vi "Two_neuron_oscillator_modulated.vi"() -> ()   [LabVIEW 2016]
uses:
  <vilib>/measure/NI_MABase.lvlib
panel:
  in  "frequency":dbl=0.625 format="%#_13g"
  out "W":T1(graph)
  in  "M":dbl[](array[numeric])=[1.0, 1.0, 1.0, -1.0, 1.0]
  in  "Simulation delay":u32=10
  out "Neurons":T2(graph)
  out "Viewer":T3={"NoPre"=[0, 2, 2], "Pre IDs"=[0, 1, 2, 1, 2], "W"=[1.0, 1.0, 1.0, -1.0, 1.0], "Current"=[1.0, 0.0, 0.0]}
  in  "stop":bool
  in  "Network AER Vectors":T3={"NoPre"=[0, 2, 2], "Pre IDs"=[0, 1, 2, 1, 2], "W"=[1.0, 1.0, 1.0, -1.0, 1.0], "Current"=[1.0, 0.0, 0.0]}
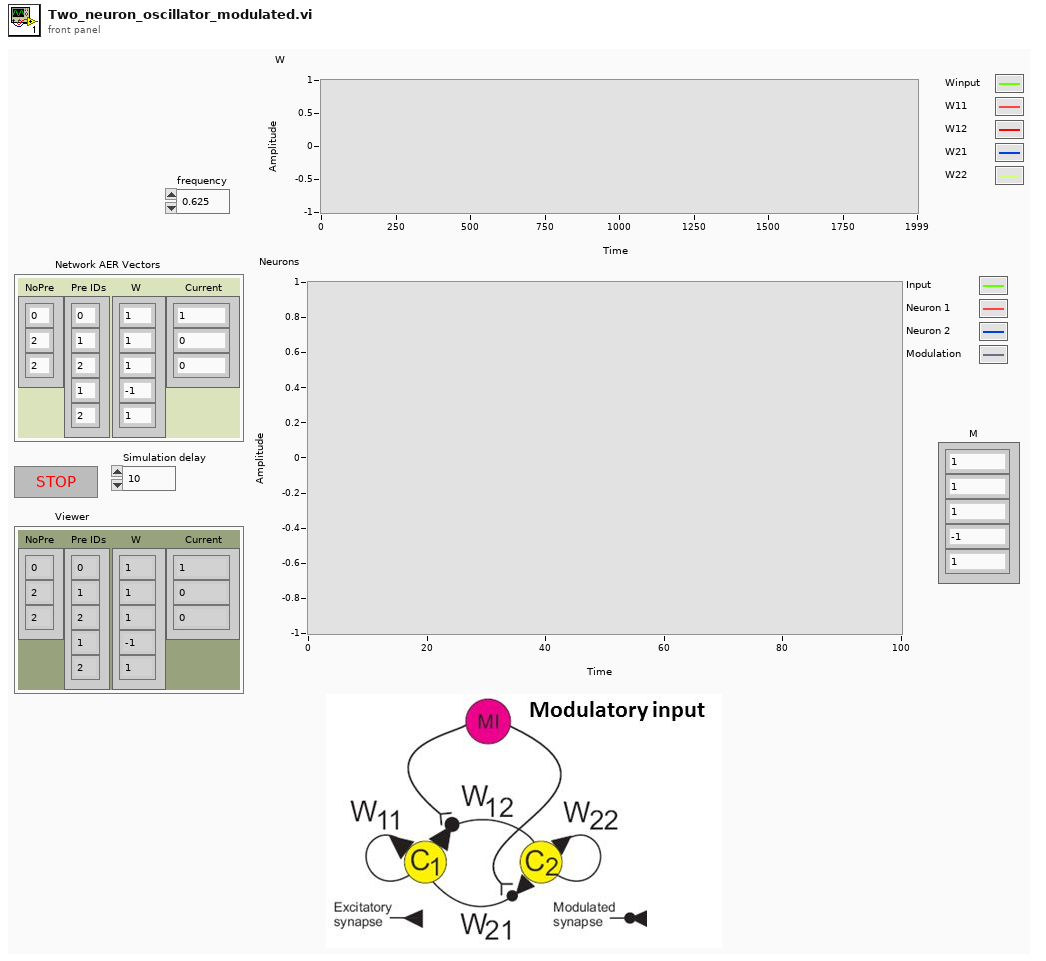
[diagram p1: front panel]
types:
  T1 = cluster{"W[0]":dbl, "W[1]":dbl, "W[2]":dbl, "W[3]":dbl, "W[4]":dbl}
  T2 = cluster{"Current[0]":dbl, "Current[1]":dbl, "Current[2]":dbl, "Current[3]":dbl}
  T3 = cluster{"NoPre":i32[], "Pre IDs":i32[], "W":dbl[], "Current":dbl[]}
  T4 = cluster{"[0]":dbl, "[1]":dbl, "[2]":dbl, "[3]":dbl}
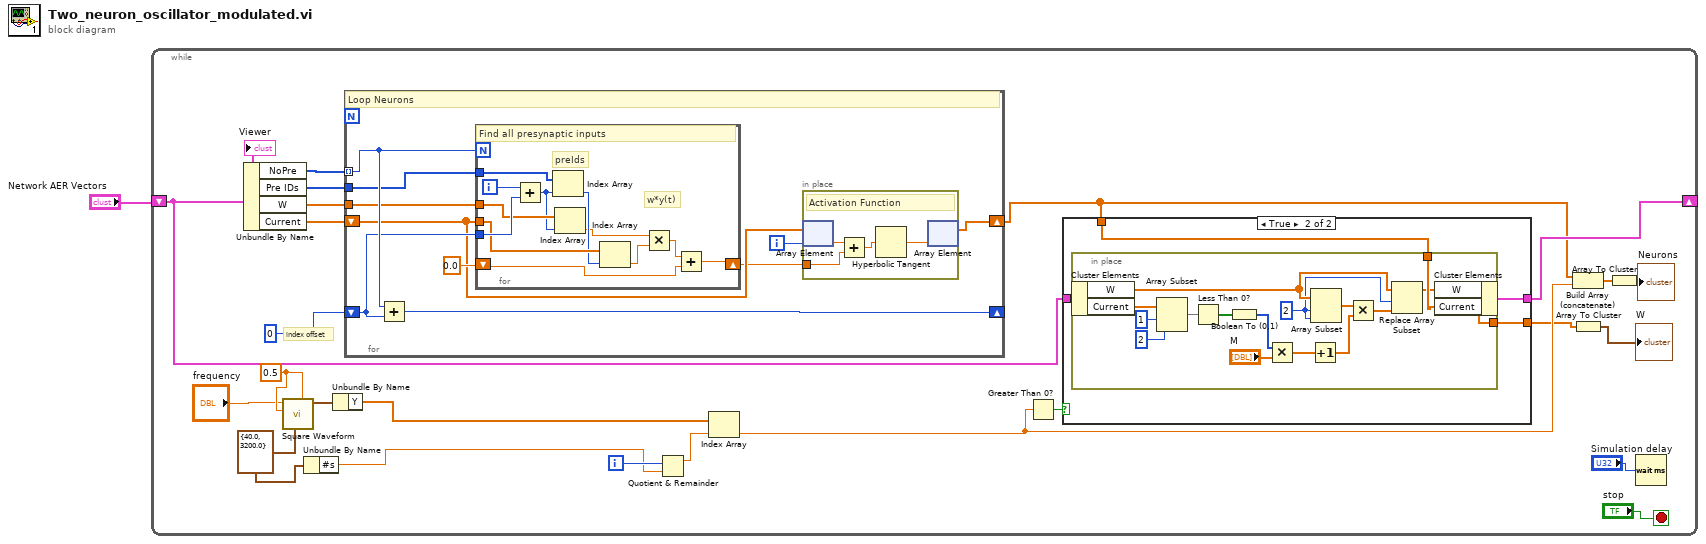
[diagram p0: block diagram]
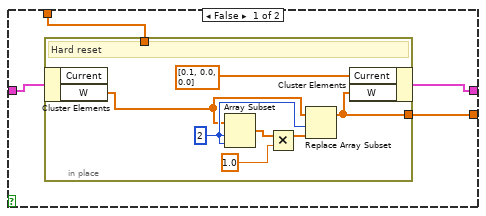
[diagram p2: hidden frame]
diagram:
  n1 = while {
    shift-right: [w11] -> _
    shift-left: "Network AER Vectors" -> [w13]
    i -> [w15]
    stop <- "stop" stop-if-true
    w7 = 0.5 ("offset")
    w6 = cluster{"Fs":dbl, "#s":dbl} {"Fs"=40.0, "#s"=3200.0} ("sampling info")
    # "index offset"
    n2 = Unbundle By Name(w13) -> ("NoPre"=w25:i32[], "Pre IDs"=w23:i32[], "W"=w22:dbl[], "Current"=w21:dbl[])
    n3 = call <vilib>:"Square Waveform.vi"("offset"=w7, "sampling info"=w6, "amplitude"=w7, "frequency"="frequency") -> ("signal out"=w5:waveform(dbl))  [unwired: 6 in, 1 out]
    n4 = Unbundle By Name(w6) -> ("#s"=w2:dbl)
    n5 = Unbundle By Name(w5) -> ("Y"=w3:dbl[])
    n6 = for {
      tunnel: w25 -> [w64] mode=indexing
      shift-right: [w65] -> _
      shift-left: 0 -> [w63]
      tunnel: w23 -> [w62]
      tunnel: w22 -> [w56]
      shift-right: [w57] -> w10
      shift-left: w21 -> [w60]
      i -> [w59]
      # "Loop Neurons"
      n7 = Add(x=w64, y=w63) -> (x+y=w65:i32)
      n8 = for {
        N: w64 -> [_]
        tunnel: w63 -> [w80]
        tunnel: w62 -> [w79]
        tunnel: w56 -> [w78]
        tunnel: w60 -> [w77]
        shift-right: [w73] -> w58
        shift-left: 0.0 -> [w71]
        i -> [w81]
        # "w*y(t)"
        # "preIds"
        # "Find all presynaptic inputs"
        n9 = Add(x=w81, y=w80) -> (x+y=w70:i32)
        n10 = Index Array(array=w79, index=w70) -> (element=w76:i32)
        n11 = Index Array(array=w78, index=w70) -> (element=w75:dbl)
        n12 = Index Array(array=w77, index=w76) -> (element=w74:dbl)
        n13 = Multiply(x=w75, y=w74) -> (x*y=w72:dbl)
        n14 = Add(x=w72, y=w71) -> (x+y=w73:dbl)
      }
      n15 = in-place {
        in-place-border: w58 -> [w69]
        # "Activation Function"
        n16 = in-place-array #1(w60, w59) -> (w67:dbl)
        n17 = Add(x=w67, y=w69) -> (x+y=w66:dbl)
        n18 = Hyperbolic Tangent(1:w66) -> (0:w68:dbl)
        n19 = in-place-array #1(w68) -> (w57:dbl[])  [unwired: 1 out]
      }
    }
    n20 = Quotient & Remainder(x=w15, y=w2) -> (x-y*floor(x/y)=w16:dbl)  [unwired: 1 out]
    n21 = Index Array(array=w3, index=w16) -> (element=w14:dbl)
    n22 = Greater Than 0?(x=w14) -> (x > 0?=w12:bool)
    n23 = case shown="True" w12 {
      tunnel: w13 -> [w29 w40]
      tunnel: [w28 w39] -> w11
      tunnel: w10 -> [w27 w38]
      tunnel: [w26 w37] -> w9
      frame False {
        n24 = in-place {
          in-place-border: w27 -> [_]
          in-place-border: [w31] -> w26
          w36 = 2 ("index")
          # "Hard reset"
          n25 = in-place-cluster #2(w29) -> ("W"=w35:dbl[])  [unwired: 1 out]
          n26 = Array Subset(array=w35, index=w36, length=w36) -> (w34:dbl[])
          n27 = Multiply(x=w34, y=1.0 ("element")) -> (x*y=w33:dbl[])
          n28 = Replace Array Subset(array=w35, new element=w33, index=w36) -> (w31:dbl[])
          n29 = in-place-cluster #2("Current"=dbl[] [0.1, 0.0, 0.0], "W"=w31) -> (w28:T3)
        }
      }
      frame True {
        n30 = in-place {
          in-place-border: w38 -> [w42]
          in-place-border: [w41] -> w37
          w46 = 2 ("index")
          n31 = in-place-cluster #3(w40) -> ("W"=w47:dbl[], "Current"=w53:dbl[])
          n32 = Array Subset(array=w53, index=1, length=2) -> (w45:dbl[])
          n33 = Less Than 0?(x=w45) -> (x < 0?=w55:bool[])
          n34 = Boolean To (0,1)(Boolean=w55) -> (0, 1=w54:i16[])
          n35 = Multiply(x=w54, y="M") -> (x*y=w52:dbl[])
          n36 = Increment(x=w52) -> (x+1=w51:dbl[])
          n37 = Array Subset(array=w47, index=w46, length=w46) -> (w49:dbl[])
          n38 = Multiply(x=w49, y=w51) -> (x*y=w48:dbl[])
          n39 = Replace Array Subset(array=w47, new element=w48, index=w46) -> (w41:dbl[])
          n40 = in-place-cluster #3("W"=w41, "Current"=w42) -> (w39:T3)
        }
      }
    }
    n41 = Build Array (concatenate)(w10, w14) -> (w17:dbl[])
    n42 = Array To Cluster(array=w9) -> (cluster=→"W":T1)
    n43 = Array To Cluster(array=w17) -> (cluster=→"Neurons":T4)
    n44 = Wait (ms)(milliseconds to wait="Simulation delay") -> ()  [unwired: 1 out]
    "Viewer" <- w13
  }
